vi "Client TX Loop.vi"(8 "error in (no error)":errorcluster, 11 "TCPMessaging in":refnum<class "TCPMessaging.lvclass">) -> (0 "error out":errorcluster)   [LabVIEW 2020, in "Vecto.lvlib" / "TCPMessaging.lvclass"]
uses:
  TCPMessaging.lvclass
  TCPMessaging.lvclass/TCPMessaging.ctl
  EventLoggingService/EventLoggingService.lvclass
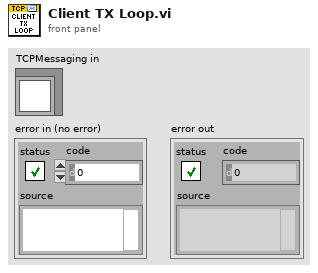
[diagram p1: front panel]
types:
  T1 = typedef "Vecto.lvlib/Send Message Data.ctl" = cluster{"TcpPayload":T2, "Register Reply":bool, "Reply Promise":refnum<class "Promise.lvclass">, "Reply Deadline":dbl}
  T2 = typedef "TcpPayload.lvlib/Data.ctl" = cluster{"target_node":u32, "source_id":u32, "sequence":u32, "timestamp":i64, "type":string, "task_id":string, "payload":u8[]}
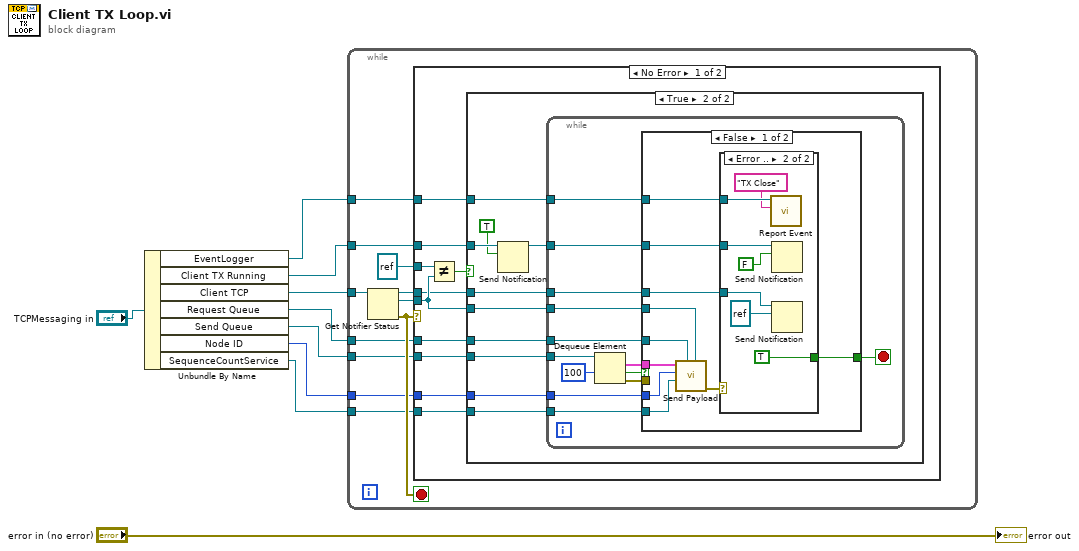
[diagram p0: block diagram]
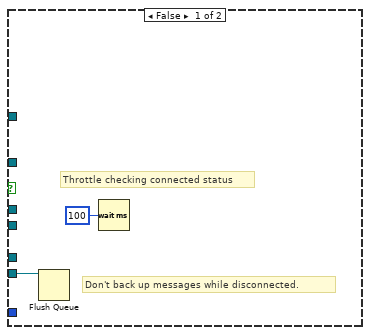
[diagram p2: hidden frame]
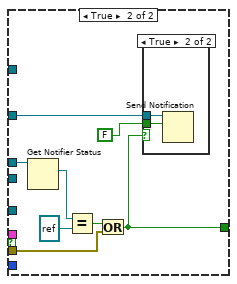
[diagram p4: hidden frame]
diagram:
  n1 = Unbundle By Name("TCPMessaging in") -> ("EventLogger"=w1:refnum<class "EventLoggingService.lvclass">, "Client TX Running"=w7:refnum<notifier>, "Client TCP"=w6:refnum<notifier>, "Request Queue"=w5:refnum<queue>, "Send Queue"=w4:refnum<queue>, "Node ID"=w3:u32, "SequenceCountService"=w2:refnum<class "SequenceCountService.lvclass">)
  n2 = while {
    tunnel: w6 -> [w20]
    tunnel: w7 -> [w16]
    tunnel: w5 -> [w14]
    tunnel: w4 -> [w13]
    tunnel: w3 -> [w12]
    tunnel: w2 -> [w11]
    tunnel: w1 -> [w10]
    stop <- w18 stop-if-true
    n3 = Get Notifier Status(notifier=w20) -> (notifier out=w15:refnum<notifier>, current notification=w19:refnum<k5>, error out=w18:errorcluster)  [unwired: 1 in, 2 out]
    n4 = case shown="No Error" w18 {
      tunnel: w19 -> [w28 _]
      tunnel: refnum<k5> refnum ("x") -> [w30 _]
      tunnel: w16 -> [w27 _]
      tunnel: w15 -> [w26 _]
      tunnel: w14 -> [w25 _]
      tunnel: w13 -> [w24 _]
      tunnel: w12 -> [w23 _]
      tunnel: w11 -> [w22 _]
      tunnel: w10 -> [w21 _]
      frame No Error {
        n5 = Not Equal?(x=w30, y=w28) -> (x != y?=w29:bool)
        n6 = case shown="True" w29 {
          tunnel: w28 -> [_ w35]
          tunnel: w27 -> [_ w42]
          tunnel: w26 -> [_ w40]
          tunnel: w25 -> [_ w39]
          tunnel: w24 -> [w32 w38]
          tunnel: w23 -> [_ w37]
          tunnel: w22 -> [_ w36]
          tunnel: w21 -> [_ w33]
          frame False {
            # "Throttle checking connected status"
            # "Don't back up messages while disconnected."
            n7 = Flush Queue(queue=w32) -> ()  [unwired: 1 in, 3 out]
            n8 = Wait (ms)(milliseconds to wait=u32 100) -> ()  [unwired: 1 out]
          }
          frame True {
            n9 = Send Notification(notification=TRUE, notifier=w42) -> (notifier out=w34:refnum<notifier>)  [unwired: 1 in, 1 out]
            n10 = while {
              tunnel: w38 -> [w54]
              tunnel: w40 -> [w49]
              tunnel: w37 -> [w52]
              tunnel: w36 -> [w51]
              tunnel: w39 -> [w50]
              tunnel: w35 -> [w46]
              tunnel: w34 -> [w45]
              tunnel: w33 -> [w43]
              stop <- w44 stop-if-true
              n11 = Dequeue Element(queue=w54, timeout in ms (-1)=100) -> (element=w53:T1, timed out?=w47:bool, error out=w55:errorcluster)  [unwired: 1 in, 1 out]
              n12 = case shown="False" w47 {
                tunnel: w55 -> [_ w76]
                tunnel: w53 -> [w65 _]
                tunnel: w52 -> [w64 _]
                tunnel: w51 -> [w63 _]
                tunnel: w50 -> [w62 _]
                tunnel: w49 -> [w61 w80]
                tunnel: w46 -> [w60 _]
                tunnel: w45 -> [w59 w75]
                tunnel: [w57 w74] -> w44
                tunnel: w43 -> [w56 _]
                frame False {
                  n13 = call "Send Payload.vi"("TCP in"=w60, "Request Queue"=w62, "SequenceCountService in"=w63, "source_id"=w64, "Send Message Data"=w65) -> ("error out"=w58:errorcluster)  [unwired: 6 in]
                  n14 = case shown="Error .." w58 {
                    tunnel: w61 -> [_ w72]
                    tunnel: w59 -> [_ w69]
                    tunnel: [_ TRUE] -> w57
                    tunnel: w56 -> [_ w67]
                    frame No Error {
                    }
                    frame Error {
                      n15 = call "Report Event.vi"("Message"="TX Close", "EventLoggingService in"=w67) -> ()  [unwired: 8 in, 2 out]
                      n16 = Send Notification(notification=FALSE, notifier=w69) -> ()  [unwired: 1 in, 2 out]
                      n17 = Send Notification(notification=refnum<k5> refnum, notifier=w72) -> ()  [unwired: 1 in, 2 out]
                    }
                  }
                }
                frame True {
                  n18 = Get Notifier Status(notifier=w80) -> (current notification=w79:refnum<k5>)  [unwired: 1 in, 4 out]
                  n19 = Equal?(x=w79, y=refnum<k5> refnum ("x")) -> (x = y?=w77:bool)
                  n20 = Or(x=w77, y=w76) -> (x .or. y?=w74:bool)
                  n21 = case shown="True" w74 {
                    tunnel: w75 -> [_ w82]
                    tunnel: FALSE -> [_ w81]
                    frame False {
                    }
                    frame True {
                      n22 = Send Notification(notification=w81, notifier=w82) -> ()  [unwired: 1 in, 2 out]
                    }
                  }
                }
              }
            }
          }
        }
      }
      frame Error {
        # "Notifier has been released, shutting down."
      }
    }
  }
  "error out" <- "error in (no error)"
